vi "WaitForMaster.vi"() -> (0 "Master There?":bool)   [LabVIEW 2016]
doc: "Checks connection with master"
uses:
  _ROSDefinition.vi
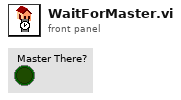
[diagram p1: front panel]
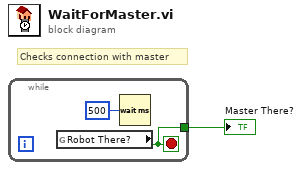
[diagram p0: block diagram]
diagram:
  # "Checks connection with master"
  n1 = while {
    tunnel: [w2] -> w1
    stop <- w2 stop-if-true
    n2 = global read "_ROSDefinition.vi" "Robot There?"() -> (w2:bool)
    n3 = Wait (ms)(milliseconds to wait=u32 500) -> ()  [unwired: 1 out]
  }
  "Master There?" <- w1
